vi "hse-application_SystemConfiguration_ReadFile.vi"(8 "error in":errorcluster, 10 "Config File":path, 11 "hse-application in":refnum<class "hse-application.lvclass">) -> (0 "error out":errorcluster, 3 "hse-application out":refnum<class "hse-application.lvclass">)   [LabVIEW 2022 SP3, in "hse-application.lvclass"]
doc: "Reads configuration parameters from the <b>Config File</b>.\n\n____\nHAMPEL SOFTWARE ENGINEERING v3.8.0 (2023-12-18 14:41)"
uses:
  hse-application.lvclass
  hse-application.lvclass/hse-application.ctl
  hse-configuration/config-ini/config-ini.lvclass
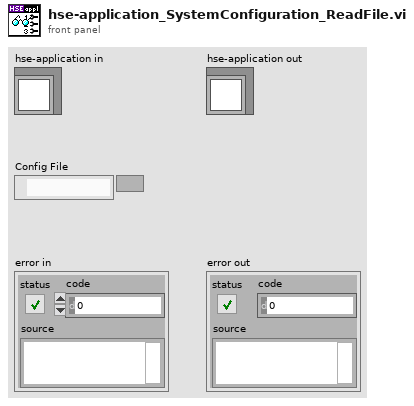
[diagram p1: front panel]
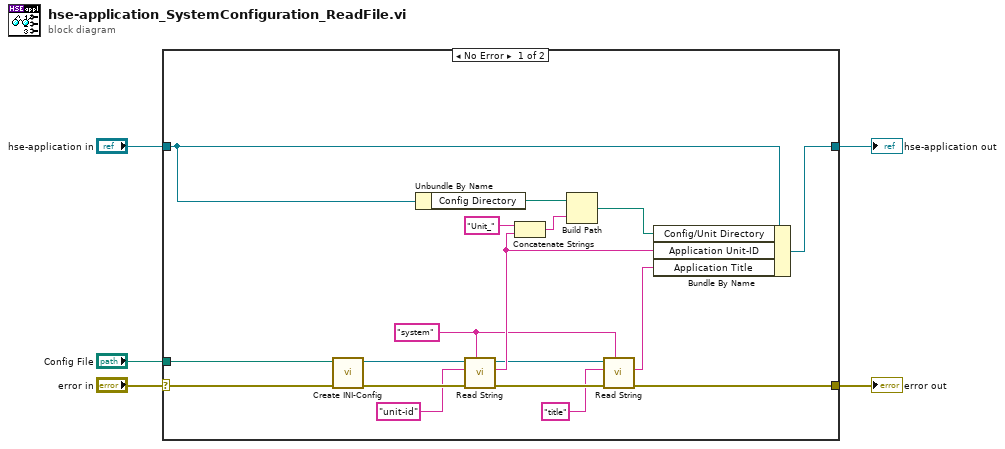
[diagram p0: block diagram]
diagram:
  n1 = case shown="No Error" "error in" {
    selector: "error in" -> [w21 w25]
    tunnel: "hse-application in" -> [w19 w24]
    tunnel: "Config File" -> [w8 _]
    tunnel: [w23 w25] -> w5
    tunnel: [w9 w24] -> w1
    frame No Error {
      w6 = "system" ("Section")
      n2 = call "Create INI-Config.vi"("error in"=w21, "INI Filepath"=w8) -> ("error out"=w20:errorcluster, "config-ini out"=w7:refnum<class "config-ini.lvclass">)  [unwired: 8 in]
      n3 = Unbundle By Name(w19) -> ("Config Directory"=w18:path)
      n4 = call-dynamic "Read String.vi"("Section"=w6, "error in"=w20, "Key"="unit-id", "config-base in"=w7) -> ("error out"=w22:errorcluster, "Value"=w16:string, "config-base out"=w15:refnum<class "config-ini.lvclass">)  [unwired: 5 in]
      n5 = Concatenate Strings("Unit_" ("name or relative path"), w16) -> (w11:string)
      n6 = Build Path(base path=w18, name or relative path=w11) -> (appended path=w12:path)
      n7 = call-dynamic "Read String.vi"("Section"=w6, "error in"=w22, "Key"="title", "config-base in"=w15) -> ("error out"=w23:errorcluster, "Value"=w17:string)  [unwired: 5 in, 1 out]
      n8 = Bundle By Name(cluster=w19, "Config/Unit Directory"=w12, "Application Unit-ID"=w16, "Application Title"=w17) -> (w9:refnum<class "hse-application.lvclass">)
    }
    frame Error {
    }
  }
  "error out" <- w5
  "hse-application out" <- w1
